vi "InterpretLoop.vi"(5 "Structure in":refnum<class "Structure.lvclass">, 6 "error in":errorcluster, 9 "VI Interpreter in":refnum<class "VI Interpreter.lvclass">) -> (0 "error out":errorcluster, 3 "VI Interpreter out":refnum<class "VI Interpreter.lvclass">, 4 "Structure out":refnum<class "Structure.lvclass">)   [LabVIEW 2014, in "VI Interpreter.lvclass"]
uses:
  VI Interpreter.lvclass
  Structure/Structure.lvclass
  Loop/Loop.lvclass
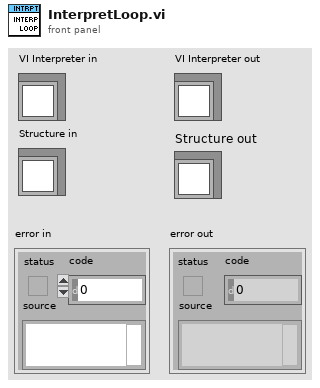
[diagram p1: front panel]
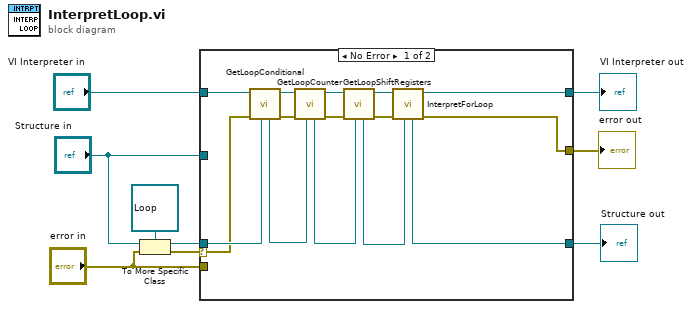
[diagram p0: block diagram]
diagram:
  n1 = To More Specific Class(target class=refnum<class "Loop.lvclass"> refnum ("Loop in"), reference="Structure in", error in="error in") -> (specific class reference=w4:refnum<class "Loop.lvclass">, error out=w3:errorcluster)
  n2 = case shown="No Error" w3 {
    selector: w3 -> [w19 _]
    tunnel: "VI Interpreter in" -> [w24 w26]
    tunnel: [w18 w25] -> w8
    tunnel: [w16 w26] -> w7
    tunnel: [w17 w27] -> w6
    tunnel: w4 -> [w20 _]
    tunnel: "error in" -> [_ w27]
    tunnel: "Structure in" -> [_ w25]
    frame No Error {
      n3 = call "GetLoopConditional.vi"("Loop in"=w20, "error in"=w19, "VI Interpreter in"=w24) -> ("error out"=w23:errorcluster, "VI Interpreter out"=w22:refnum<class "VI Interpreter.lvclass">, "Loop out"=w21:refnum<class "Loop.lvclass">)  [unwired: 4 in]
      n4 = call "GetLoopCounter.vi"("Loop in"=w21, "error in"=w23, "VI Interpreter in"=w22) -> ("error out"=w13:errorcluster, "VI Interpreter out"=w15:refnum<class "VI Interpreter.lvclass">, "Loop out"=w11:refnum<class "Loop.lvclass">)  [unwired: 4 in]
      n5 = call "GetLoopShiftRegisters.vi"("Loop in"=w11, "error in"=w13, "VI Interpreter in"=w15) -> ("error out"=w12:errorcluster, "VI Interpreter out"=w14:refnum<class "VI Interpreter.lvclass">, "Loop out"=w10:refnum<class "Loop.lvclass">)  [unwired: 4 in]
      n6 = call "InterpretForLoop.vi"("Loop in"=w10, "error in"=w12, "VI Interpreter in"=w14) -> ("error out"=w17:errorcluster, "VI Interpreter out"=w16:refnum<class "VI Interpreter.lvclass">, "Loop out"=w18:refnum<class "Loop.lvclass">)  [unwired: 4 in]
    }
    frame Error {
    }
  }
  "error out" <- w6
  "VI Interpreter out" <- w7
  "Structure out" <- w8
